vi "recalc_shunt_values.vi"(1 "DFTBins":u16[](array[numeric])=[1, 2, 3, 7, 11, 17, 23, 31, 43, 61, 89, 127, 179, 251, 349], 2 "DIV":u32(ring)=1 items=["1"=1, "2"=2, "4"=4, "6"=6, "8"=8, "10"=10, "12"=12, "14"=14, "16"=16, "20"=20, "24"=24, "28"=28, "32"=32, "40"=40, "48"=48, "56"=56, "64"=64, "80"=80, "96"=96, "112"=112, "128"=128, "160"=160, "192"=192, "196"=196, "224"=224, "256"=256, "320"=320, "384"=384, "448"=448, "512"=512, "640"=640, "768"=768, "896"=896, "1024"=1024, "1280"=1280, "1536"=1536, "1792"=1792], 3 "FE_shunt_data":sgl[](array[numeric]), 5 "error in (no error)":errorcluster) -> (11 "Frequencies":string, 15 "shunt":cdb[](array[numeric]), 17 "freqs":dbl[](array[numeric]), 19 "error out":errorcluster)   [LabVIEW 2017, in "ZBOX_IS.lvlib"]
uses:
  ZBOX_IS.lvlib
  <vilib>/Analysis/NI_AALPro.lvlib
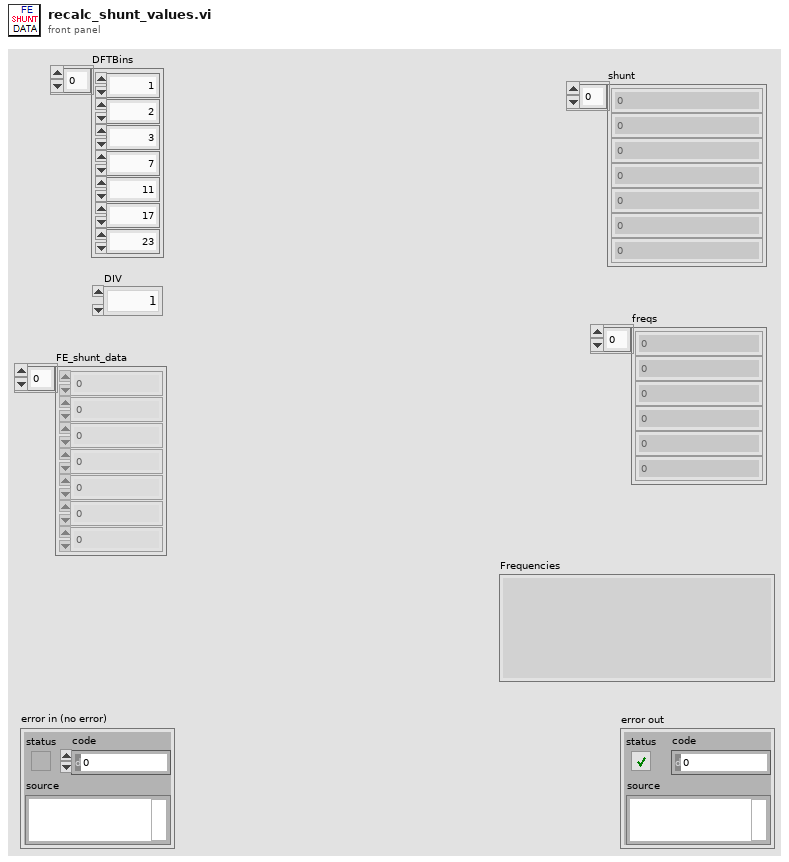
[diagram p1: front panel]
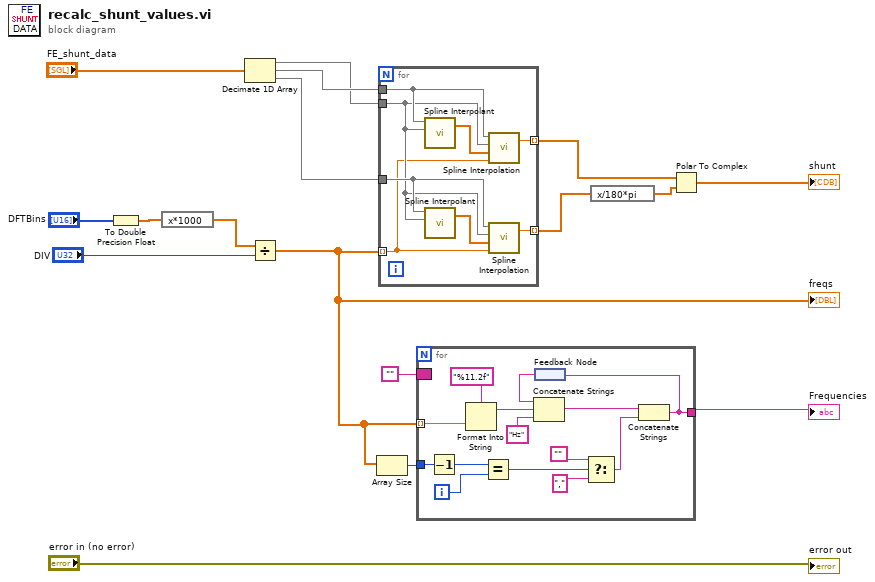
[diagram p0: block diagram]
diagram:
  n1 = To Double Precision Float(number="DFTBins") -> (double precision float=w13:dbl[])
  n2 = expression code="x*1000"(w13) -> (w12:dbl[])
  n3 = Decimate 1D Array("FE_shunt_data") -> (w14:sgl[], w16:sgl[], w15:sgl[])
  n4 = Divide(x=w12, y="DIV") -> (x/y=w2:dbl[])
  "freqs" <- w2
  n5 = Array Size(array=w2) -> (size(s)=w4:i32)
  n6 = for {
    tunnel: w16 -> [w25]
    tunnel: w14 -> [w19]
    tunnel: w2 -> [w18] mode=indexing
    tunnel: [w23] -> w8 mode=indexing
    tunnel: w15 -> [w20]
    tunnel: [w22] -> w7 mode=indexing
    n7 = call <vilib>:"Spline Interpolant.vi"("X"=w19, "Y"=w25) -> ("Interpolant"=w24:dbl[])  [unwired: 2 in, 1 out]
    n8 = call <vilib>:"Spline Interpolant.vi"("X"=w19, "Y"=w20) -> ("Interpolant"=w21:dbl[])  [unwired: 2 in, 1 out]
    n9 = call <vilib>:"Spline Interpolation.vi"("x value"=w18, "Interpolant"=w24, "X"=w19, "Y"=w25) -> ("interpolation value"=w23:dbl)  [unwired: 1 out]
    n10 = call <vilib>:"Spline Interpolation.vi"("x value"=w18, "Interpolant"=w21, "X"=w19, "Y"=w20) -> ("interpolation value"=w22:dbl)  [unwired: 1 out]
  }
  n11 = for {
    tunnel: w2 -> [w39] mode=indexing
    border: "" -> [_]
    tunnel: [w33] -> w1
    tunnel: w4 -> [w32]
    i -> [w31]
    n12 = Decrement(x=w32) -> (x-1=w26:i32)
    n13 = Format Into String(format string="%11.2f", w39) -> (resulting string=w38:string)  [unwired: 2 in, 1 out]
    n14 = Equal?(x=w26, y=w31) -> (x = y?=w29:bool)
    n15 = feedback #1() -> (w37:string)
    n16 = Concatenate Strings(w37, w38, "Hz" ("string")) -> (w34:string)
    n17 = Select(t="", s=w29, f="," ("string")) -> (s? t:f=w28:string)
    n18 = Concatenate Strings(w34, w28) -> (w33:string)
    n19 = feedback-in #1(w33) -> ()
  }
  "Frequencies" <- w1
  n20 = expression code="x/180*pi"(w7) -> (w9:dbl[])
  n21 = Polar To Complex(1:w9, 2:w8) -> (0:→"shunt":cdb[])
  "error out" <- "error in (no error)"
